vi "Interactive Demo.vi"() -> ()   [LabVIEW 2013, in "dotNETChart XControl.xctl"]
uses:
  dotNETChart XControl.xctl
  typedefs/3DSettings.ctl
  <vilib>/express/express shared/transition.llb/Dynamic To Waveform Array.vi
  <vilib>/express/express signal manip/GetorSetDDTAttributes/Set DDT Attributes/SetT0.vi
  <vilib>/express/express shared/transition.llb/Waveform Array To Dynamic.vi
  <vilib>/express/express signal manip/GetorSetDDTAttributes/Set DDT Attributes/Set DDT Properties.xnode
panel:
  in  "Chart Type 2":i32(ring)=4 caption="Chart Type"
  in  "Series 1 Data Colour":u32(colorbox)=6836 caption="Series Data Colour"
  in  "series name":string="First Series Title" caption="xaxislabel"
  in  "Chart Palette":u16(ring)
  in  "Chart Type":i32(ring)=4
  in  "Chart Wall Gradient Colour":u32(colorbox)=12116479
  in  "Gradient Style":i32(ring)=4
  in  "Chart Wall Border Colour":u32(colorbox)=16777238
  in  "Chart Wall Colour":u32(colorbox)
  in  "chart_wall_trans":u8(slide)=31 caption="Chart Wall Opacity" scale=0.0..255.0
  in  "Legend Style":u16(ring) items=["Column", "Row", "Table"]
  in  "Mouse Zoom":u16(ring)=1 items=["off", "on (2D mode only)"]
  in  "Series 2 Data Colour":u32(colorbox)=12116479 caption="Series Data Colour"
  in  "Skin Style":i32(ring)=1 items=["None", "Emboss", "Raised", "Sunken", "FrameThin1", "FrameThin2", "FrameThin3", "FrameThin4", "FrameThin5", "FrameThin6", "FrameTitle1", "FrameTitle2", "FrameTitle3", "FrameTitle4", "FrameTitle5", "FrameTitle6", "FrameTitle7", "FrameTitle8"]
  in  "yaxislabel":string="Y axis label" caption="xaxislabel"
  in  "xaxislabel":string="X axis label"
  in  "3dmode":bool=TRUE caption="3D Mode"
  in  "Rotation":i32=25
  in  "Wall Width":i32=2
  in  "Perspective":i32=4
  in  "LightStyle":i32(ring)=2 items=["None", "Simplistic", "Realistic"]
  in  "Inclination":i32=21
  in  "Random":bool
  out "dotNETChart XControl":dynamicdata(xcontrol)=[{"t0"=timestamp(3359225754.779551 s since 1904-01-01), "dt"=0.001, "Y"=[-0.21293878372691832, 0.10480719171607178, 0.5198645121842703, 0.4960927860135643, 0.8486500407057044, -0.19156178243419908, -0.3213988951228298, -1.0007275322775073, -1.3720240757016509, -0.2660093892305525, -0.23724681626115568, 0.796814395938406, 0.9778645666014882, 0.7870343306028441, 0.7585739928106939, 0.26409213430431566, -0.8946529385336436, -1.169162891258134, -1.1556662975978256, -0.3690681531689127], "attributes"=variant("NI_ChannelName"=variant(string "First Series Title"), "NI_ExpIsRelativeTime"=variant(bool FALSE), "NI_ExpStartTimeStamp"=variant(timestamp timestamp(3359225754.779551 s since 1904-01-01)), "NI_ExpTimeStamp"=variant(timestamp timestamp(3359225754.779551 s since 1904-01-01)), "NI_ExpXDimension"=variant(string "t"))}, {"t0"=timestamp(3359225754.779551 s since 1904-01-01), "dt"=0.001, "Y"=[-0.22651223041771185, 0.4171889778375242, 0.6017245565566697, 0.9588615672567297, 0.748101089941119, -0.27993796654087566, -0.8863552944000307, -1.0635191133061586, -0.9344284949437466, -0.1710474405944974, 0.3018910917348227, 0.5301156955284767, 1.4475242535659825, 1.1713473149513396, 0.25407740207025176, -0.025061984573477407, -0.48652113815437137, -0.7534989399164532, -1.2184058505207012, -0.10043002227520204], "attributes"=variant("NI_ChannelName"=variant(string "Sine with Uniform Noise"), "NI_ExpIsRelativeTime"=variant(bool FALSE), "NI_ExpStartTimeStamp"=variant(timestamp timestamp(3359225754.779551 s since 1904-01-01)), "NI_ExpTimeStamp"=variant(timestamp timestamp(3359225754.779551 s since 1904-01-01)), "NI_ExpXDimension"=variant(string "t"))}]
  # "Settings"
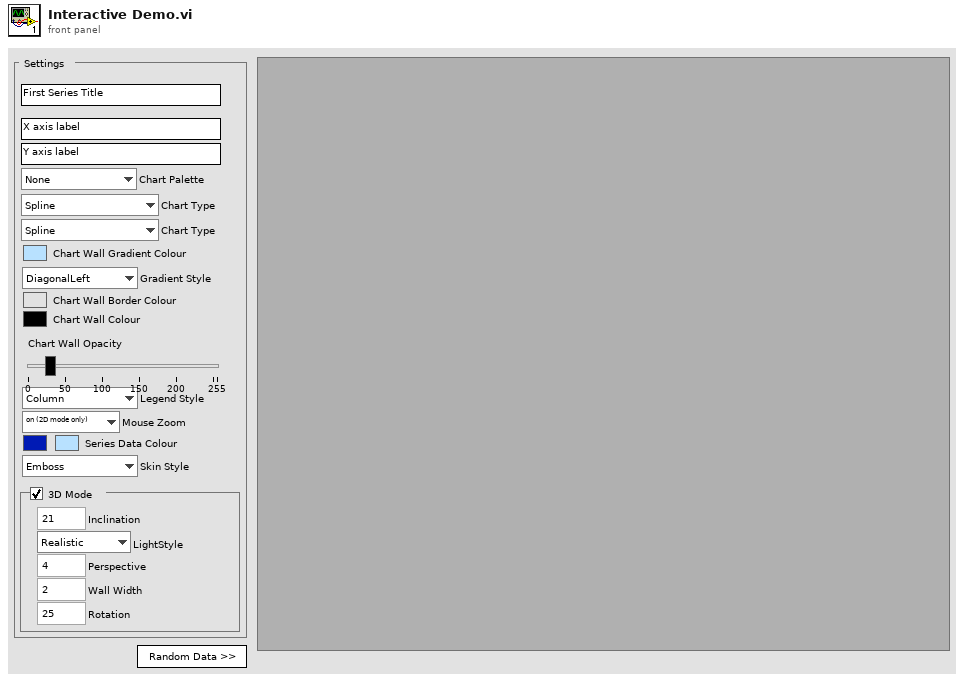
[diagram p1: front panel]
types:
  T1 = typedef "ChartType.ctl" = i32
  T2 = typedef "BackGradientStyle.ctl" = i32
  T3 = typedef "LegendStyle.ctl" = i32
  T4 = typedef "SkinStyle.ctl" = i32
  T5 = typedef "3DSettings.ctl" = cluster{"Inclination":i32, "LightStyle":i32, "Perspective":i32, "WallWidth":i32, "Rotation":i32}
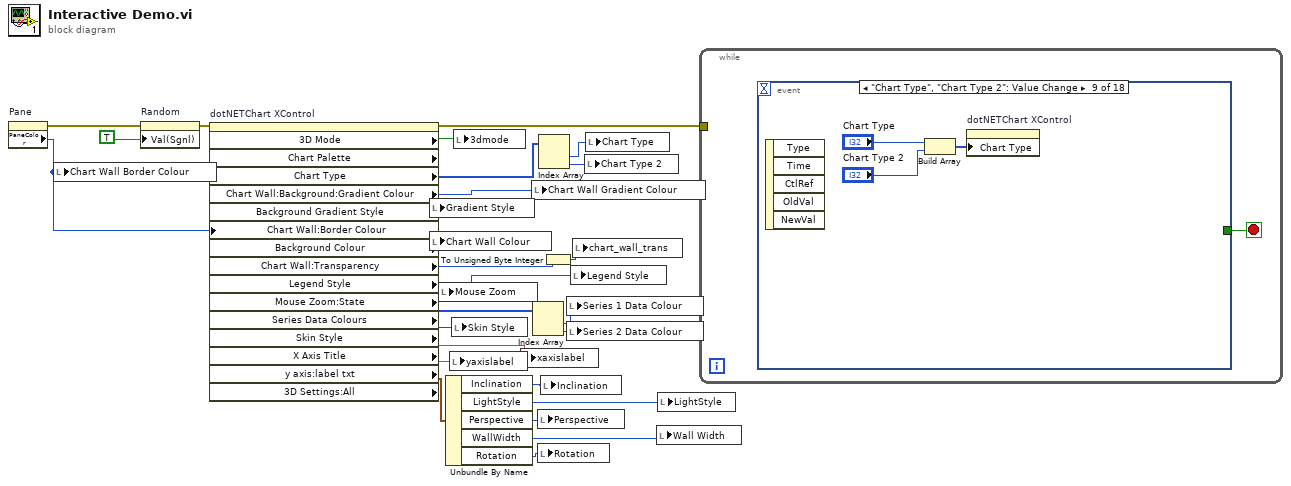
[diagram p0: block diagram]
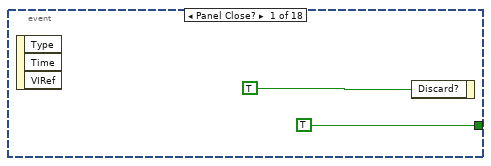
[diagram p2: hidden frame]
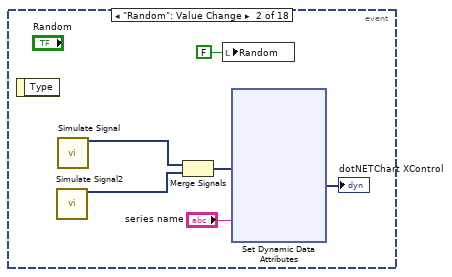
[diagram p3: hidden frame]
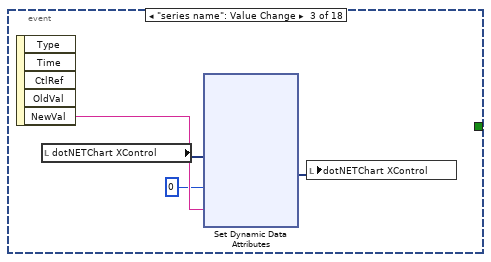
[diagram p4: hidden frame]
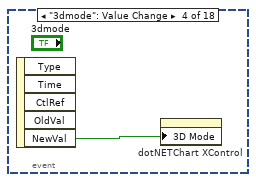
[diagram p5: hidden frame]
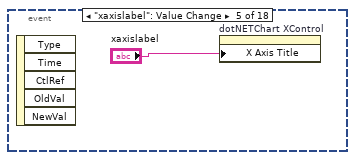
[diagram p6: hidden frame]
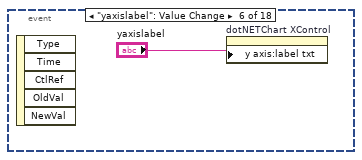
[diagram p7: hidden frame]
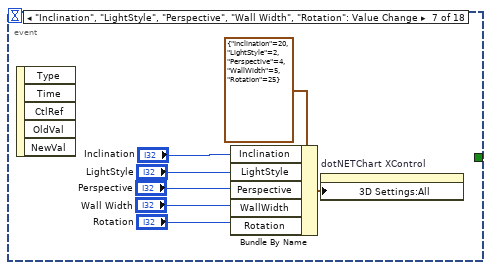
[diagram p8: hidden frame]
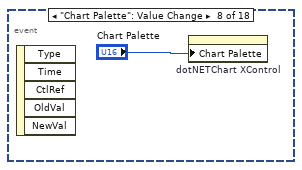
[diagram p9: hidden frame]
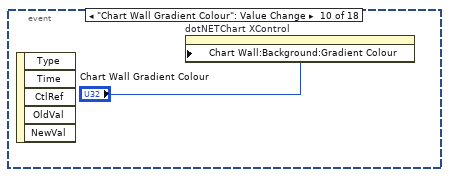
[diagram p10: hidden frame]
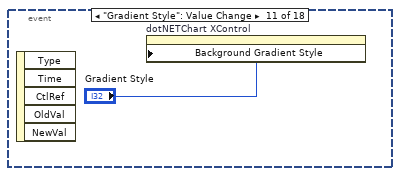
[diagram p11: hidden frame]
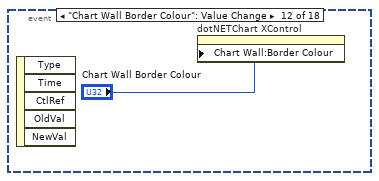
[diagram p12: hidden frame]
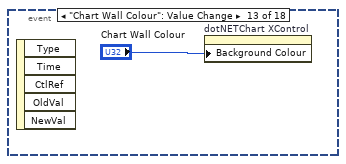
[diagram p13: hidden frame]
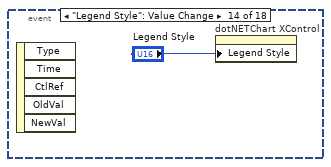
[diagram p14: hidden frame]
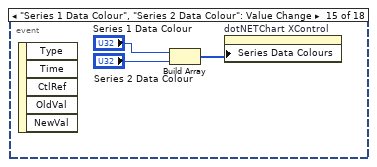
[diagram p15: hidden frame]
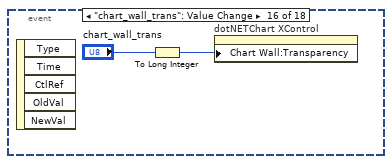
[diagram p16: hidden frame]
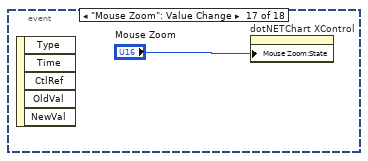
[diagram p17: hidden frame]
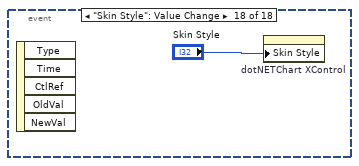
[diagram p18: hidden frame]
diagram:
  n1 = property on="Pane" class="Pane"() -> (error out=w4:errorcluster, "PaneColor"=w5:u32)  [unwired: 2 in, 1 out]
  n2 = local write "Chart Wall Border Colour"(w5) -> ()
  n3 = property on="Random" class="Bool (strict)"(error in=w4, "Val(Sgnl)"=TRUE ("Random")) -> (error out=w27:errorcluster)  [unwired: 1 in, 1 out]
  n4 = property on="dotNETChart XControl" class="dotNETChart XControl (strict)" props=["3D Mode", "Chart Palette", "Chart Type", "Chart Wall:Background:Gradient Colour", "Background Gradient Style", "Chart Wall:Border Colour", "Background Colour", "Chart Wall:Transparency", "Legend Style", "Mouse Zoom:State", "Series Data Colours", "Skin Style", "X Axis Title", "y axis:label txt", "3D Settings:All"](error in=w27, "Chart Wall:Border Colour"=w5) -> (error out=w26:errorcluster, "3D Mode"=w25:bool, "Chart Type"=w7:T1[], "Chart Wall:Background:Gradient Colour"=w8:u32, "Background Gradient Style"=w9:T2, "Background Colour"=w11:u32, "Chart Wall:Transparency"=w10:i32, "Legend Style"=w13:T3, "Mouse Zoom:State"=w14:enum16{"off", "on (2D mode only)"}, "Series Data Colours"=w15:u32[], "Skin Style"=w16:T4, "X Axis Title"=w18:string, "y axis:label txt"=w17:string, "3D Settings:All"=w24:T5)  [unwired: 1 in, 2 out]
  n5 = local write "Gradient Style"(w9) -> ()
  n6 = local write "Chart Wall Colour"(w11) -> ()
  n7 = local write "Mouse Zoom"(w14) -> ()
  n8 = Unbundle By Name(w24) -> ("Inclination"=w23:i32, "LightStyle"=w22:i32, "Perspective"=w21:i32, "WallWidth"=w20:i32, "Rotation"=w19:i32)
  n9 = local write "yaxislabel"(w17) -> ()
  n10 = local write "Skin Style"(w16) -> ()
  n11 = local write "3dmode"(w25) -> ()
  n12 = local write "xaxislabel"(w18) -> ()
  n13 = local write "Chart Wall Gradient Colour"(w8) -> ()
  n14 = Index Array(array=w15) -> (element #1=w2:u32, element #2=w3:u32)  [unwired: 2 in]
  n15 = local write "Perspective"(w21) -> ()
  n16 = local write "Rotation"(w19) -> ()
  n17 = Index Array(array=w7) -> (element #1=w6:T1, element #2=w1:T1)  [unwired: 2 in]
  n18 = local write "Inclination"(w23) -> ()
  n19 = To Unsigned Byte Integer(number=w10) -> (unsigned 8bit integer=w12:u8)
  n20 = local write "Series 1 Data Colour"(w2) -> ()
  n21 = local write "Series 2 Data Colour"(w3) -> ()
  n22 = local write "Legend Style"(w13) -> ()
  n23 = local write "chart_wall_trans"(w12) -> ()
  n24 = local write "Chart Type 2"(w1) -> ()
  n25 = local write "Chart Type"(w6) -> ()
  n26 = local write "Wall Width"(w20) -> ()
  n27 = local write "LightStyle"(w22) -> ()
  n28 = while {
    tunnel: w26 -> [_]
    stop <- w29 stop-if-true
    n29 = event shown="[8] \"Chart Type\", \"Chart Type 2\": Value Change" {
      selector: _ -> [_ _ _ _ _ _ _ _ _ _ _ _ _ _ _ _ _ _]
      dyn-events: _ -> [_ _ _ _ _ _ _ _ _ _ _ _ _ _ _ _ _ _]
      timeout: _ -> [_ _ _ _ _ _ _ _ _ _ _ _ _ _ _ _ _ _]
      tunnel: [TRUE _ _ _ _ _ _ _ _ _ _ _ _ _ _ _ _ _] -> w29
      event Panel Close? {
        n30 = event-data() -> ()  [unwired: 1 in, 3 out]
        n31 = event-data("Discard?"=TRUE) -> ()  [unwired: 1 in, 1 out]
      }
      event "Random": Value Change {
        n32 = event-data() -> ()  [unwired: 1 in, 1 out]
        n33 = call "Simulate Signal2"() -> ("Sine with Uniform Noise"=w32:dynamicdata)  [unwired: 14 in, 1 out]
        n34 = call "Simulate Signal"() -> ("Sine with Uniform Noise"=w37:dynamicdata)  [unwired: 14 in, 1 out]
        n35 = Merge Signals(w37, w32) -> (w33:dynamicdata)
        n36 = local write "Random"(FALSE ("Random")) -> ()
        n37 = xnode "Set Dynamic Data Attributes"("Signals In"=w33, "Signal Name"="series name") -> ("Signals Out"=→"dotNETChart XControl":dynamicdata)  [unwired: 2 in, 1 out]
      }
      event "series name": Value Change {
        n38 = event-data() -> ("NewVal"=w53:string)  [unwired: 1 in, 4 out]
        n39 = local read "dotNETChart XControl"() -> (w54:dynamicdata)
        n40 = xnode "Set Dynamic Data Attributes"("Signals In"=w54, "Signal Index"=0, "Signal Name"=w53) -> ("Signals Out"=w55:dynamicdata)  [unwired: 1 in, 1 out]
        n41 = local write "dotNETChart XControl"(w55) -> ()
      }
      event "3dmode": Value Change {
        n42 = event-data() -> ("NewVal"=w69:bool)  [unwired: 1 in, 4 out]
        n43 = property on="dotNETChart XControl" class="dotNETChart XControl (strict)"("3D Mode"=w69) -> ()  [unwired: 2 in, 2 out]
      }
      event "xaxislabel": Value Change {
        n44 = event-data() -> ()  [unwired: 1 in, 5 out]
        n45 = property on="dotNETChart XControl" class="dotNETChart XControl (strict)"("X Axis Title"="xaxislabel") -> ()  [unwired: 2 in, 2 out]
      }
      event "yaxislabel": Value Change {
        n46 = event-data() -> ()  [unwired: 1 in, 5 out]
        n47 = property on="dotNETChart XControl" class="dotNETChart XControl (strict)"("y axis:label txt"="yaxislabel") -> ()  [unwired: 2 in, 2 out]
      }
      event "Inclination", "LightStyle", "Perspective", "Wall Width", "Rotation": Value Change {
        n48 = event-data() -> ()  [unwired: 1 in, 5 out]
        n49 = Bundle By Name(cluster=T5 {"Inclination"=20, "LightStyle"=2, "Perspective"=4, "WallWidth"=5, "Rotation"=25} ("3D Settings:All Elements"), "Inclination"="Inclination", "LightStyle"="LightStyle", "Perspective"="Perspective", "WallWidth"="Wall Width", "Rotation"="Rotation") -> (w77:T5)
        n50 = property on="dotNETChart XControl" class="dotNETChart XControl (strict)"("3D Settings:All"=w77) -> ()  [unwired: 2 in, 2 out]
      }
      event "Chart Palette": Value Change {
        n51 = event-data() -> ()  [unwired: 1 in, 5 out]
        n52 = property on="dotNETChart XControl" class="dotNETChart XControl (strict)"("Chart Palette"="Chart Palette") -> ()  [unwired: 2 in, 2 out]
      }
      event "Chart Type", "Chart Type 2": Value Change {
        n53 = event-data() -> ()  [unwired: 1 in, 5 out]
        n54 = Build Array("Chart Type", "Chart Type 2") -> (w82:i32[])
        n55 = property on="dotNETChart XControl" class="dotNETChart XControl (strict)"("Chart Type"=w82) -> ()  [unwired: 2 in, 2 out]
      }
      event "Chart Wall Gradient Colour": Value Change {
        n56 = event-data() -> ()  [unwired: 1 in, 5 out]
        n57 = property on="dotNETChart XControl" class="dotNETChart XControl (strict)"("Chart Wall:Background:Gradient Colour"="Chart Wall Gradient Colour") -> ()  [unwired: 2 in, 2 out]
      }
      event "Gradient Style": Value Change {
        n58 = event-data() -> ()  [unwired: 1 in, 5 out]
        n59 = property on="dotNETChart XControl" class="dotNETChart XControl (strict)"("Background Gradient Style"="Gradient Style") -> ()  [unwired: 2 in, 2 out]
      }
      event "Chart Wall Border Colour": Value Change {
        n60 = event-data() -> ()  [unwired: 1 in, 5 out]
        n61 = property on="dotNETChart XControl" class="dotNETChart XControl (strict)"("Chart Wall:Border Colour"="Chart Wall Border Colour") -> ()  [unwired: 2 in, 2 out]
      }
      event "Chart Wall Colour": Value Change {
        n62 = event-data() -> ()  [unwired: 1 in, 5 out]
        n63 = property on="dotNETChart XControl" class="dotNETChart XControl (strict)"("Background Colour"="Chart Wall Colour") -> ()  [unwired: 2 in, 2 out]
      }
      event "Legend Style": Value Change {
        n64 = event-data() -> ()  [unwired: 1 in, 5 out]
        n65 = property on="dotNETChart XControl" class="dotNETChart XControl (strict)"("Legend Style"="Legend Style") -> ()  [unwired: 2 in, 2 out]
      }
      event "Series 1 Data Colour", "Series 2 Data Colour": Value Change {
        n66 = event-data() -> ()  [unwired: 1 in, 5 out]
        n67 = Build Array("Series 1 Data Colour", "Series 2 Data Colour") -> (w90:u32[])
        n68 = property on="dotNETChart XControl" class="dotNETChart XControl (strict)"("Series Data Colours"=w90) -> ()  [unwired: 2 in, 2 out]
      }
      event "chart_wall_trans": Value Change {
        n69 = event-data() -> ()  [unwired: 1 in, 5 out]
        n70 = To Long Integer(number="chart_wall_trans") -> (32bit integer=w91:i32)
        n71 = property on="dotNETChart XControl" class="dotNETChart XControl (strict)"("Chart Wall:Transparency"=w91) -> ()  [unwired: 2 in, 2 out]
      }
      event "Mouse Zoom": Value Change {
        n72 = event-data() -> ()  [unwired: 1 in, 5 out]
        n73 = property on="dotNETChart XControl" class="dotNETChart XControl (strict)"("Mouse Zoom:State"="Mouse Zoom") -> ()  [unwired: 2 in, 2 out]
      }
      event "Skin Style": Value Change {
        n74 = event-data() -> ()  [unwired: 1 in, 5 out]
        n75 = property on="dotNETChart XControl" class="dotNETChart XControl (strict)"("Skin Style"="Skin Style") -> ()  [unwired: 2 in, 2 out]
      }
    }
  }
